vi "Create Link.vi"(4 "Style":T1={"Width"=1, "Style"=enum."Solid"}, 6 "Color":u32(colorbox), 7 "Selectable":bool=TRUE, 8 "error in (no error)":errorcluster, 9 "Destination":refnum<data-value>, 10 "Source":refnum<data-value>) -> (0 "error out":errorcluster, 3 "Link Reference":refnum<data-value>)   [LabVIEW 2017, in "LV Image Editor Framework.lvlib" / "Link.lvclass"]
uses:
  Link.lvclass
  Shape/Shape.lvclass
  C:/Github/LIEF/Forms/Shape/Shape.lvclass
  C:/Github/LIEF/Forms/Line/Line.lvclass
  Link.lvclass/Link.ctl
  Shape/Shape.lvclass/Shape.ctl
  Line/Line.lvclass/Line.ctl
  Shape/Write Color.vi
  Shape/Write Movable.vi
  Line/Write Style.vi
  Shape/Write Selectable.vi
  Selection/Selection.lvclass
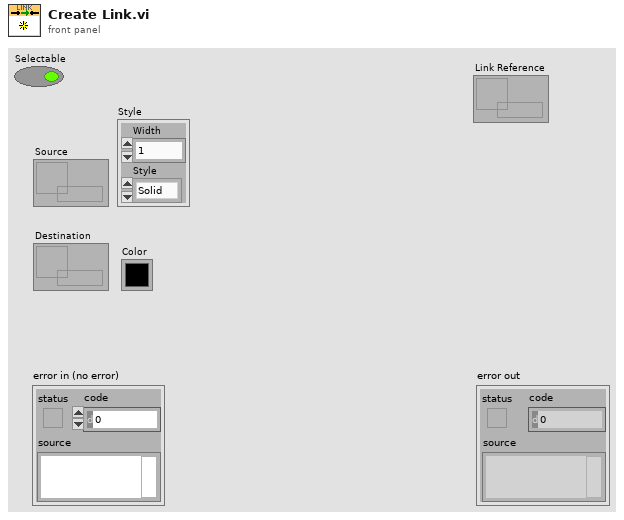
[diagram p1: front panel]
types:
  T1 = cluster{"Width":u16, "Style":enum32{"Solid", "Dash", "Dot", "DashDot", "DashDotDot"}}
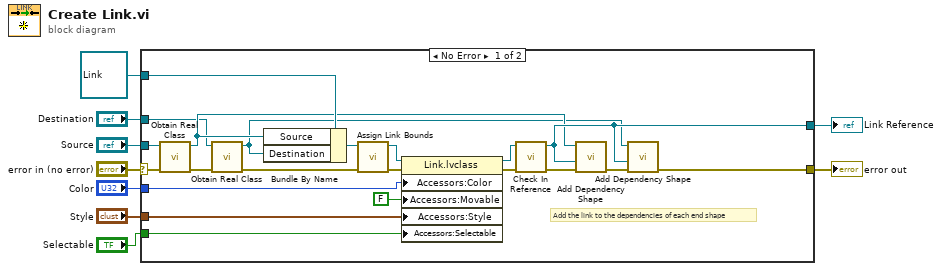
[diagram p0: block diagram]
diagram:
  n1 = case shown="No Error" "error in (no error)" {
    selector: "error in (no error)" -> [w12 w31]
    tunnel: [w22 w31] -> w8
    tunnel: refnum<class "Link.lvclass"> refnum ("Link in") -> [w25 _]
    tunnel: "Source" -> [w16 _]
    tunnel: "Destination" -> [w14 _]
    tunnel: [w20 _] -> w2
    tunnel: "Color" -> [w29 _]
    tunnel: "Style" -> [w28 _]
    tunnel: "Selectable" -> [w17 _]
    frame No Error {
      # "Add the link to the dependencies of each end shape"
      n2 = call "Obtain Real Class.vi"("error in (no error)"=w12, "Shape"=w16) -> ("error out"=w11:errorcluster, "Inner Shape"=w15:refnum<data-value>)  [unwired: 8 in]
      n3 = call "Obtain Real Class.vi"("error in (no error)"=w11, "Shape"=w14) -> ("error out"=w10:errorcluster, "Inner Shape"=w13:refnum<data-value>)  [unwired: 8 in]
      n4 = Bundle By Name(cluster=w25, "Source"=w15, "Destination"=w13) -> (w24:refnum<class "Link.lvclass">)
      n5 = call "Assign Link Bounds.vi"("error in (no error)"=w10, "Link in"=w24) -> ("error out"=w26:errorcluster, "Link out"=w30:refnum<class "Link.lvclass">)  [unwired: 8 in]
      n6 = property class="Link.lvclass"(reference=w30, error in=w26, "Accessors:Color"=w29, "Accessors:Movable"=FALSE ("Movable"), "Accessors:Style"=w28, "Accessors:Selectable"=w17) -> (reference out=w21:refnum<class "Link.lvclass">, error out=w19:errorcluster)
      n7 = call "Check In Reference.vi"("error in (no error)"=w19, "Shape in"=w21) -> ("error out"=w18:errorcluster, "Shape Reference"=w20:refnum<data-value>)  [unwired: 8 in]
      n8 = call "Add Dependency Shape.vi"("error in (no error)"=w18, "Dependency Shape"=w20, "Shape Ref in"=w15) -> ("error out"=w23:errorcluster)  [unwired: 7 in, 1 out]
      n9 = call "Add Dependency Shape.vi"("error in (no error)"=w23, "Dependency Shape"=w20, "Shape Ref in"=w13) -> ("error out"=w22:errorcluster)  [unwired: 7 in, 1 out]
    }
    frame Error {
    }
  }
  "error out" <- w8
  "Link Reference" <- w2
